vi "Read Array from file.vi"(4 "error in":errorcluster, 5 "bytes to read":i32, 6 "File location in":i64, 7 "File":refnum<file>) -> (0 "error out":errorcluster, 1 "Array of U8s":u8[](array[numeric]), 2 "File location after array read":i64, 3 "File out":refnum<file>)   [LabVIEW 2015, in "Tiff reader.lvlib"]
doc: "This .vi reads a section of the file and returns the U8 array."
uses:
  Tiff reader.lvlib
panel:
  out "change location?":bool
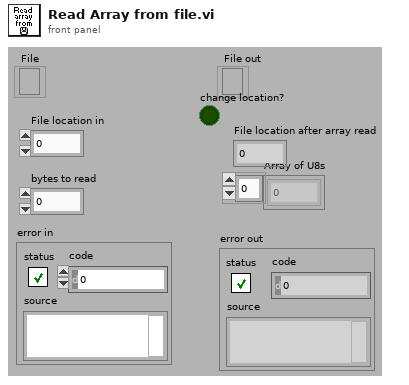
[diagram p1: front panel]
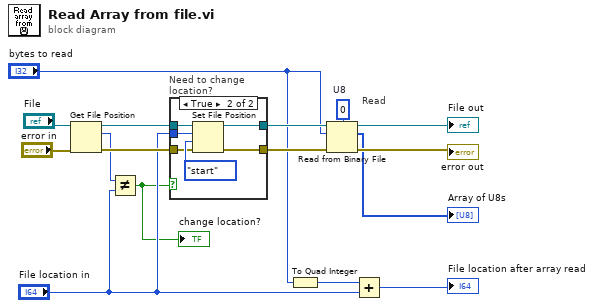
[diagram p0: block diagram]
diagram:
  w11 = u8 0  # U8
  # "Read"
  n1 = Get File Position(4:"error in", 7:"File") -> (0:w7:errorcluster, 2:w5:i64, 3:w6:refnum<file>)
  n2 = Not Equal?(x=w5, y="File location in") -> (x != y?=w3:bool)
  "change location?" <- w3
  n3 = case "Need to change location?" shown="True" w3 {
    tunnel: [w18 w24] -> w13
    tunnel: [w17 w23] -> w12
    tunnel: w7 -> [w17 w21]
    tunnel: w6 -> [w18 w20]
    tunnel: "File location in" -> [_ w19]
    frame False {
    }
    frame True {
      n4 = Set File Position(offset (in bytes) (0)=w19, refnum=w20, from (0:start)=enum16{"start", "end", "current"}."start", error in=w21) -> (refnum out=w24:refnum<file>, error out=w23:errorcluster)
    }
  }
  n5 = To Quad Integer(1:"bytes to read") -> (0:w1:i64)
  n6 = Read from Binary File(5:w11, 8:w12, 10:"bytes to read", 11:w13) -> (0:→"error out":errorcluster, 2:→"Array of U8s":u8[], 3:→"File out":refnum<file>)  [unwired: 3 out]
  n7 = Add(x=w1, y="File location in") -> (x+y=→"File location after array read":i64)
